vi "EMV T7 Flow Conditions.vi"(4 "Detection Slope":dbl=0.2 format="%#_13g", 6 "T7_DELTA_INDICATING_FLOW":dbl, 8 "error in (no error)":errorcluster, 9 "Cold Water Supply Temperature":dbl, 10 "T7_DELTA_FLOW_THRESHOLD":dbl, 11 "T7 History":dbl[](array[numeric])) -> (0 "error out":errorcluster, 2 "T7 Detect?":bool)   [LabVIEW 2016]
panel:
  out "Slope Chart":dbl(graph)
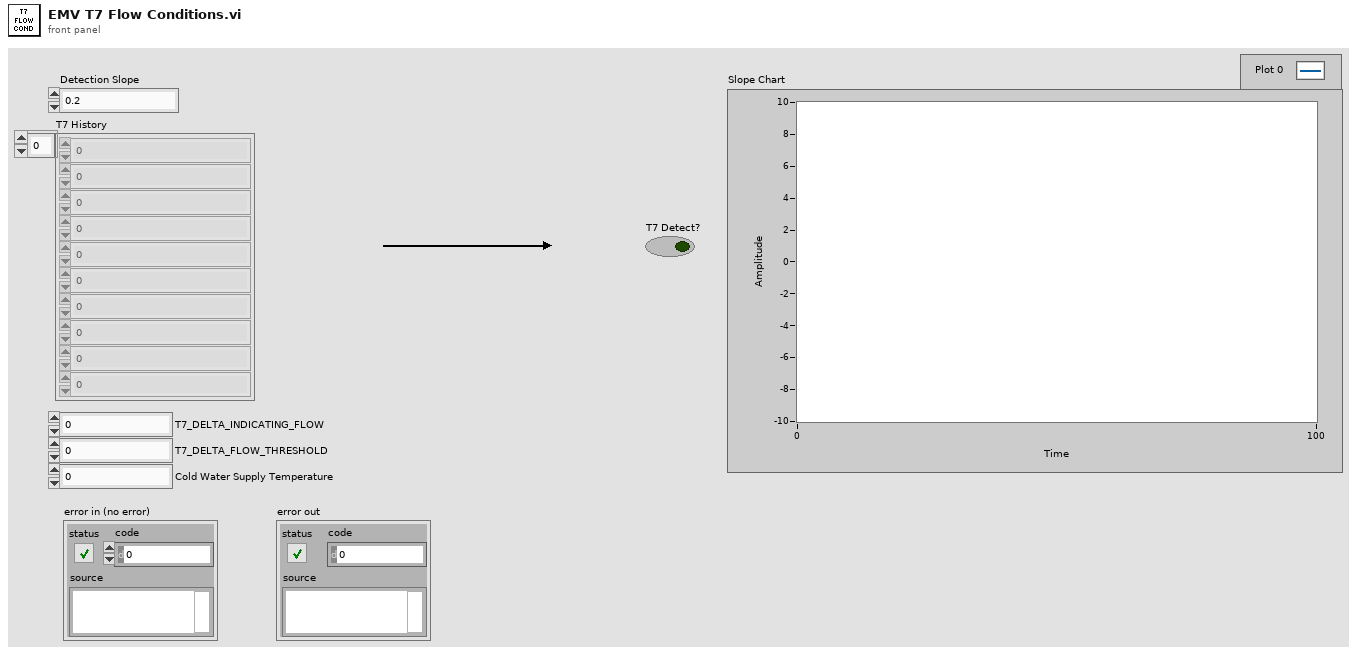
[diagram p1: front panel]
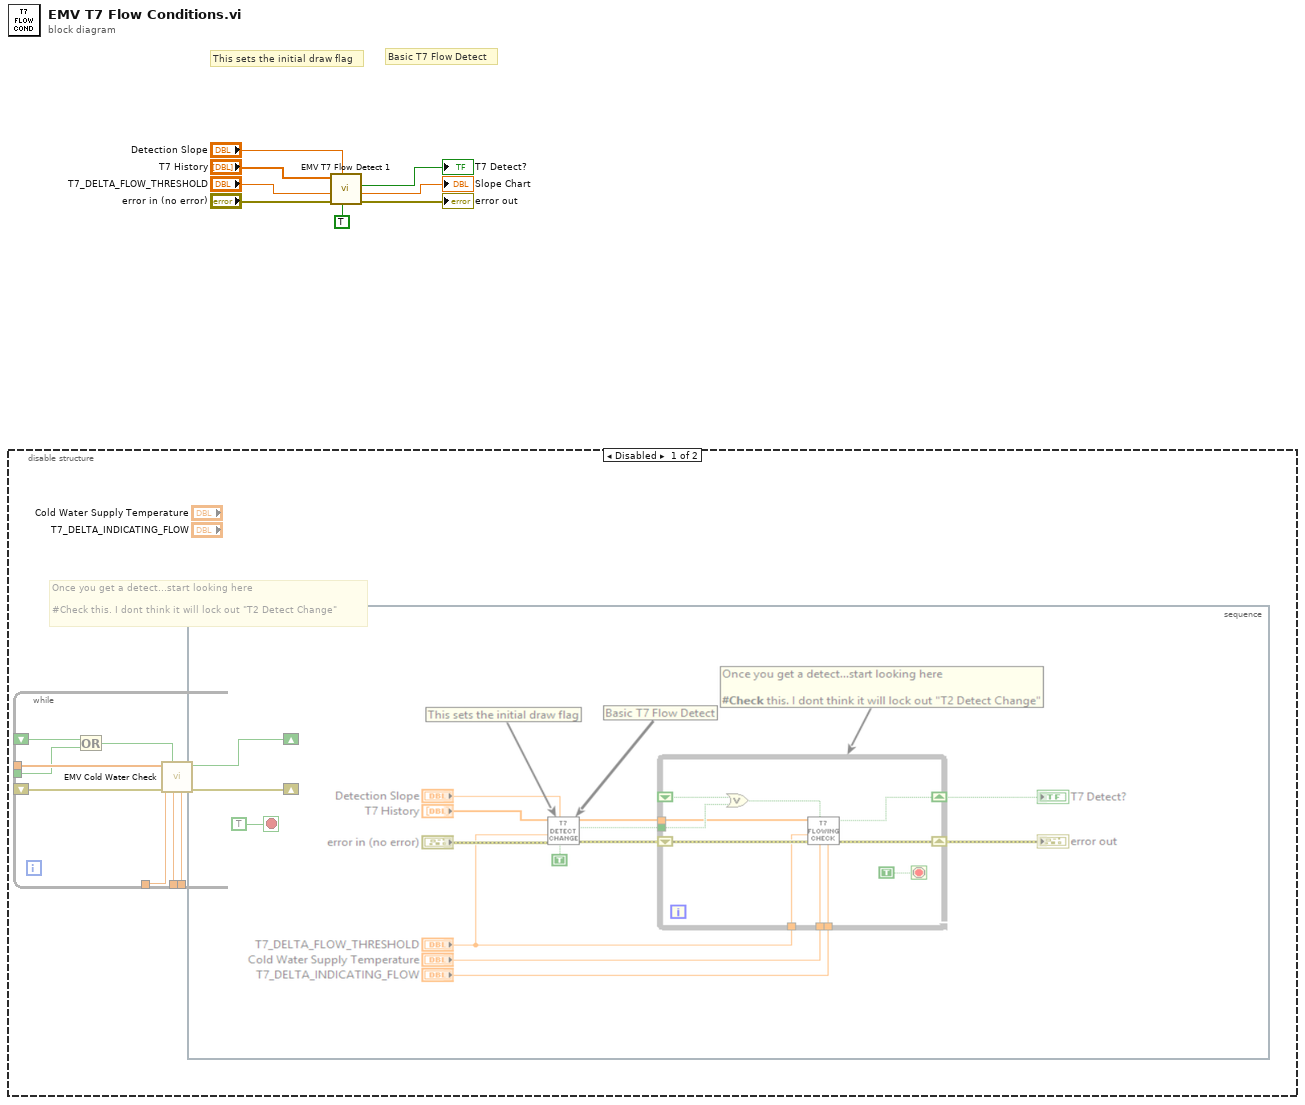
[diagram p0: block diagram]
diagram:
  # "Basic T7 Flow Detect"
  # "This sets the initial draw flag"
  n1 = disable-structure shown="Disabled" {
    frame Disabled {
      # "Once you get a detect...start looking here\n\n#Check this. I dont think it will lock out \"T2 Detect Change\""
      n2 = while {
        tunnel: _ -> [w13]
        tunnel: _ -> [w19]
        tunnel: _ -> [w18]
        tunnel: _ -> [w15]
        shift-right: [w16] -> _
        shift-left: _ -> [w12]
        shift-right: [w17] -> _
        shift-left: _ -> [w11]
        tunnel: _ -> [w10]
        stop <- TRUE stop-if-true
        n3 = Or(x=w11, y=w10) -> (x .or. y?=w9:bool)
        n4 = call "EMV Cold Water Check.vi"("T7_DELTA_INDICATING_FLOW"=w19, "Cold Water Supply Temperature"=w18, "T7 Detect?"=w9, "error in (no error)"=w12, "T7_DELTA_FLOW_THRESHOLD"=w15, "Current T7 Temperatures"=w13) -> ("error out"=w16:errorcluster, "T7 Detect?"=w17:bool)  [unwired: 4 in]
      }
      n5 = stacked-sequence {
        frame #0 {
        }
      }
    }
    frame Enabled {
    }
  }
  n6 = call "EMV T7 Flow Detect 1.vi"("Detect Flow Start?"=TRUE, "Detection Slope"="Detection Slope", "error in (no error)"="error in (no error)", "T7_DELTA_FLOW_THRESHOLD"="T7_DELTA_FLOW_THRESHOLD", "Current T7 Temperatures"="T7 History") -> ("error out"=→"error out":errorcluster, "slope"=→"Slope Chart":dbl, "Detection?"=→"T7 Detect?":bool)  [unwired: 3 in, 1 out]
